vi "acq.PL.vi"(7 "DVR":T2, 8 "error in":errorcluster) -> (0 "error out":errorcluster, 2 "Refnum out":T1, 3 "buffer":u16[][](array[numeric]))   [LabVIEW 2020]
uses:
  _controls/data.ctl
  camera/camera.lvclass
  _controls/data.ref.ctl
  <vilib>/vision/Image Controls.llb/IMAQ Image.ctl
  _controls/state.ctl
  _controls/data.vars.ctl
  _controls/save_options.ctl
  _controls/flip.ctl
  1370ff9f-c20d-4950-b9a9-0a12fa6452b0.vi
  891f7916-19d5-4c28-9165-e0da2aba2f3a.vi
  lib/O-PL.dll
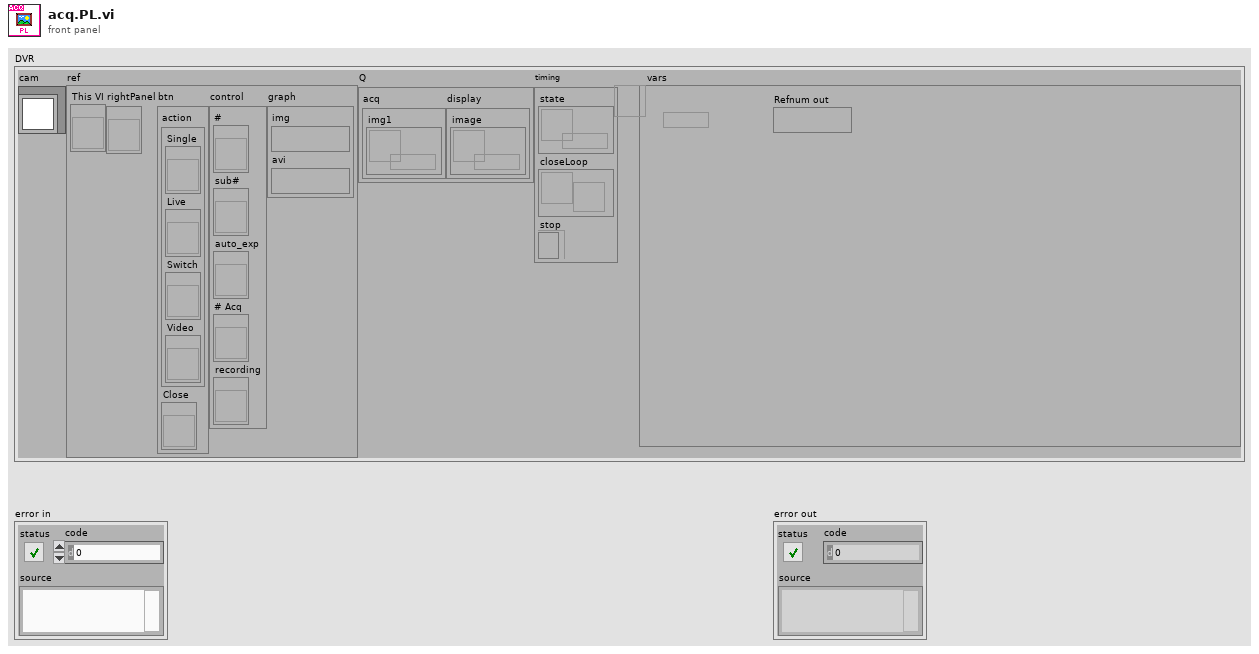
[diagram p1: front panel]
types:
  T1 = typedef "IMAQ Image.ctl" = refnum<image>
  T2 = typedef "data.ctl" = cluster{"cam":refnum<class "camera.lvclass">, "ref":T3, "Q":cluster{"acq":cluster{"img1":refnum<queue>}, "display":cluster{"image":refnum<queue>}}, "timing":cluster{"state":refnum<queue>, "closeLoop":refnum<notifier>, "stop":refnum<k4>}, "vars":refnum<data-value>}
  T3 = typedef "data.ref.ctl" = cluster{"This VI":refnum<vi>, "rightPanel":refnum<vi>, "btn":cluster{"action":cluster{"Single":refnum<vi>, "Live":refnum<vi>, "Switch":refnum<vi>, "Video":refnum<vi>}, "Close":refnum<vi>}, "control":cluster{"#":refnum<vi>, "sub#":refnum<vi>, "auto_exp":refnum<vi>, "# Acq":refnum<vi>, "recording":refnum<vi>}, "graph":cluster{"img":T1, "avi":T1}}
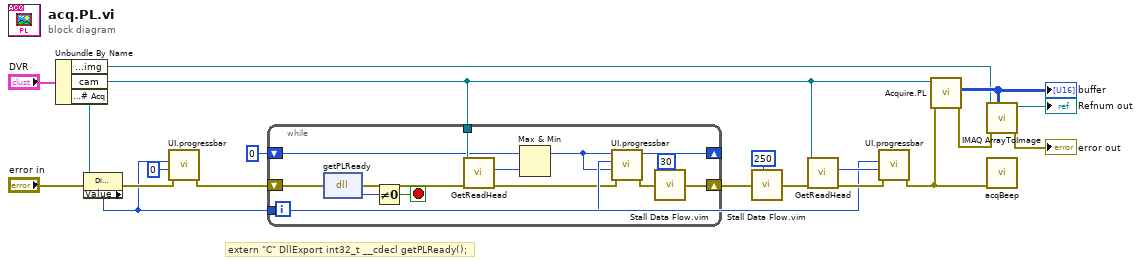
[diagram p0: block diagram]
diagram:
  # "extern \"C\" DllExport int32_t __cdecl getPLReady();"
  n1 = Unbundle By Name("DVR") -> ("ref.graph.img"=w15:T1, "cam"=w1:refnum<class "camera.lvclass">, "ref.control.# Acq"=w13:refnum<vi>)
  n2 = property class="DigNum (strict)"(reference=w13, error in="error in") -> (error out=w11:errorcluster, "Value"=w2:u64)  [unwired: 1 out]
  n3 = call "UI.progressbar.vi"("error in"=w11, "Value"=u8 0, "Maximum"=w2) -> ("error out"=w10:errorcluster)  [unwired: 8 in]
  n4 = while {
    shift-right: [w21] -> w12
    shift-left: w10 -> [w30]
    tunnel: w2 -> [w33]
    tunnel: w1 -> [w28]
    shift-right: [w24] -> _
    shift-left: u64 0 -> [w25]
    stop <- w32 stop-if-true
    n5 = dll-call lib="D:/UNSW - New/v0.8.3/lib/O-PL.dll" fn="getPLReady"(error in=w30) -> (error out=w23:errorcluster, "return"=w31:i32)  [unwired: 2 in, 1 out]
    n6 = Not Equal To 0?(x=w31) -> (x != 0?=w32:bool)
    n7 = call "GetReadHead.vi"("error in"=w23, "camera.nit_c in"=w28) -> ("error out"=w27:errorcluster, "LastImageNumber"=w26:i64)  [unwired: 8 in]
    n8 = Max & Min(x=w25, y=w26) -> (max(x,y)=w24:u64)  [unwired: 1 out]
    n9 = call "UI.progressbar.vi"("error in"=w27, "Value"=w24, "Maximum"=w33) -> ("error out"=w22:errorcluster)  [unwired: 8 in]
    n10 = call "Stall Data Flow.vim"("value in"=w22, "milliseconds to wait"=u32 30) -> ("value out"=w21:errorcluster)  [unwired: 1 out]
  }
  n11 = call "Stall Data Flow.vim"("value in"=w12, "milliseconds to wait"=u32 250) -> ("value out"=w7:errorcluster)  [unwired: 1 out]
  n12 = call "GetReadHead.vi"("error in"=w7, "camera.nit_c in"=w1) -> ("error out"=w6:errorcluster, "LastImageNumber"=w3:i64)  [unwired: 8 in]
  n13 = call "UI.progressbar.vi"("error in"=w6, "Value"=w3, "Maximum"=w2) -> ("error out"=w5:errorcluster)  [unwired: 8 in]
  n14 = call-dynamic "Acquire.PL.vi"("error in"=w5, "camera.nit in"=w1) -> ("error out"=w16:errorcluster, "buffer"=w20:u16[][])  [unwired: 8 in]
  "buffer" <- w20
  n15 = call "IMAQ ArrayToImage"("Image Pixels (U16)"=w20, "error in (no error)"=w16, "Image"=w15) -> ("error out"=→"error out":errorcluster, "Image Out"=→"Refnum out":T1)  [unwired: 7 in]
  n16 = call "acqBeep.vi"("error in"=w5) -> ()  [unwired: 10 in, 1 out]
